vi "Getting Started - External Memory (FPGA).vi"() -> ()   [LabVIEW 2023]
doc: "This VI demonstrates the different methods of accessing DRAM on a FLexRIO FPGA Module."
uses:
  <vilib>/Platform/TimedLoop/XDataNode/wakeup.ctl
  <vilib>/Platform/TimedLoop/XDataNode/XDNodeRunTimeDep.lvlib
  <vilib>/Platform/TimedLoop/XDataNode/nitl_modes.ctl
  <vilib>/Platform/TimedLoop/XDataNode/timing_clust.ctl
  <vilib>/Platform/TimedLoop/XDataNode/XDataNode.xnode
  <instrlib>/_niInstr/Basic Elements/v1/FPGA/niInstr Basic Elements v1 FPGA.lvlib
  <instrlib>/_niInstr/Memory/v1/FPGA/DRAM/niInstr Memory DRAM v1 FPGA.lvclass
  <vilib>/rvi/DataTransferAndStorage/Container/XNode/niFpgaContainer.xnode
  <vilib>/rvi/Memory/Memory_Emulation/niFpgaMemoryFastEmulationDramWriteAndRequestData.vi
  <vilib>/rvi/Memory/Memory_Emulation/niFpgaMemoryEmulationDramWriteAndRequestData.vi
  <instrlib>/_niInstr/Memory/v1/FPGA/Memory/Public/Write Data (With Byte Enables).ctl
  <instrlib>/_niInstr/Memory/v1/FPGA/Memory/niInstr Memory v1 FPGA.lvclass
  <instrlib>/_niInstr/Memory/v1/FPGA/Memory/Public/Read Request.ctl
  <instrlib>/_niInstr/Memory/v1/FPGA/DRAM/Public/Timeslot Arbiter Configuration.ctl
  <instrlib>/_niInstr/Data Formatting/v1/FPGA/niInstr Data Formatting v1 FPGA.lvlib
  <instrlib>/_niInstr/Data Formatting/v1/FPGA/Private/Convert/U64 array to Boolean Array.vi
  <instrlib>/_niInstr/Data Formatting/v1/FPGA/Private/Convert/Boolean Array to U64 Array.vi
  <instrlib>/_niInstr/Memory/v1/FPGA/DRAM U64/Public/Create.vi
  <instrlib>/_niInstr/Memory/v1/FPGA/DRAM U64/niInstr Memory DRAM U64 v1 FPGA.lvclass
  <instrlib>/_niInstr/Memory/v1/FPGA/DRAM U128/Public/Create.vi
  <instrlib>/_niInstr/Memory/v1/FPGA/DRAM U128/niInstr Memory DRAM U128 v1 FPGA.lvclass
  <instrlib>/_niInstr/Memory/v1/FPGA/DRAM U512/Public/Create.vi
  <instrlib>/_niInstr/Memory/v1/FPGA/DRAM U512/niInstr Memory DRAM U512 v1 FPGA.lvclass
  <instrlib>/_niInstr/Basic Elements/v1/FPGA/Private/Write U32 FIFO.vi
  <instrlib>/_niInstr/Basic Elements/v1/FPGA/Private/Read U32 FIFO.vi
  <instrlib>/FlexRIO/DRAM FIFO/v2/FPGA/DRAM FIFO/DRAM FIFO v2 FPGA.lvclass
  <instrlib>/FlexRIO/DRAM FIFO/v2/FPGA/DRAM FIFO/Private/DRAM FIFO U512/Create 512x1 DRAM FIFO.vi
  <instrlib>/FlexRIO/DRAM FIFO/v2/FPGA/DRAM FIFO/Private/DRAM FIFO U512/DRAM FIFO U512 v2 FPGA.lvclass
  <instrlib>/FlexRIO/DRAM FIFO/v2/FPGA/DRAM FIFO/FIFO Depth.ctl
  <instrlib>/FlexRIO/DRAM FIFO/v2/FPGA/DRAM FIFO/Private/DRAM FIFO U64/Create 64x1 DRAM FIFO.vi
  <instrlib>/FlexRIO/DRAM FIFO/v2/FPGA/DRAM FIFO/Private/DRAM FIFO U64/DRAM FIFO U64 v2 FPGA.lvclass
  <instrlib>/FlexRIO/DRAM FIFO/v2/FPGA/DRAM FIFO/Private/DRAM FIFO U128/Create 128x1 DRAM FIFO.vi
  <instrlib>/FlexRIO/DRAM FIFO/v2/FPGA/DRAM FIFO/Private/DRAM FIFO U128/DRAM FIFO U128 v2 FPGA.lvclass
  <instrlib>/FlexRIO/DRAM FIFO/v2/FPGA/DRAM FIFO/Pack U32.vi
  <instrlib>/FlexRIO/DRAM FIFO/v2/FPGA/DRAM FIFO/Unpack U8.vi
  <vilib>/rvi/Memory/Memory_Emulation/niFpgaMemoryEmulationDramRetrieveData.vi
  <instrlib>/_niInstr/Memory/v1/FPGA/DRAM U256/Public/Create.vi
  <instrlib>/_niInstr/Memory/v1/FPGA/DRAM U256/niInstr Memory DRAM U256 v1 FPGA.lvclass
  <instrlib>/FlexRIO/DRAM FIFO/v2/FPGA/DRAM FIFO/Private/DRAM FIFO U256/Create 256x1 DRAM FIFO.vi
  <instrlib>/FlexRIO/DRAM FIFO/v2/FPGA/DRAM FIFO/Private/DRAM FIFO U256/DRAM FIFO U256 v2 FPGA.lvclass
  <instrlib>/FlexRIO/DRAM FIFO/v2/FPGA/DRAM FIFO/DRAM FIFO Status.ctl
panel:
  out "DRAM FIFO Status":T1
  out "elements per valid output":i32
  in  "DRAM FIFO - read grant time":u16=100
  in  "DRAM FIFO - write grant time":u16=100
  in  "Memory IDL - Write Data":u64[](array[numeric])=[0, 0, 0, 0, 0, 0, 0, 0]
  out "Memory Primitive - Retrieved Data":u64
  in  "Memory Primitive - Request Valid":bool
  in  "Memory Primitive - Request Address":u32
  out "Memory IDL - Retrieved Data":u64[](array[numeric])
  in  "Memory IDL - read grant time":u16
  in  "Memory IDL - write grant time":u16
  in  "Memory IDL - Request Valid":bool
  in  "Memory IDL - Request Address":u32
  in  "Memory IDL - Write Valid":bool
  in  "Memory IDL - Write Address":u32
  in  "Memory Primitive - Write Valid":bool=TRUE
  in  "Memory Primitive - Write Data":u64
  in  "Memory Primitive - Write Address":u32
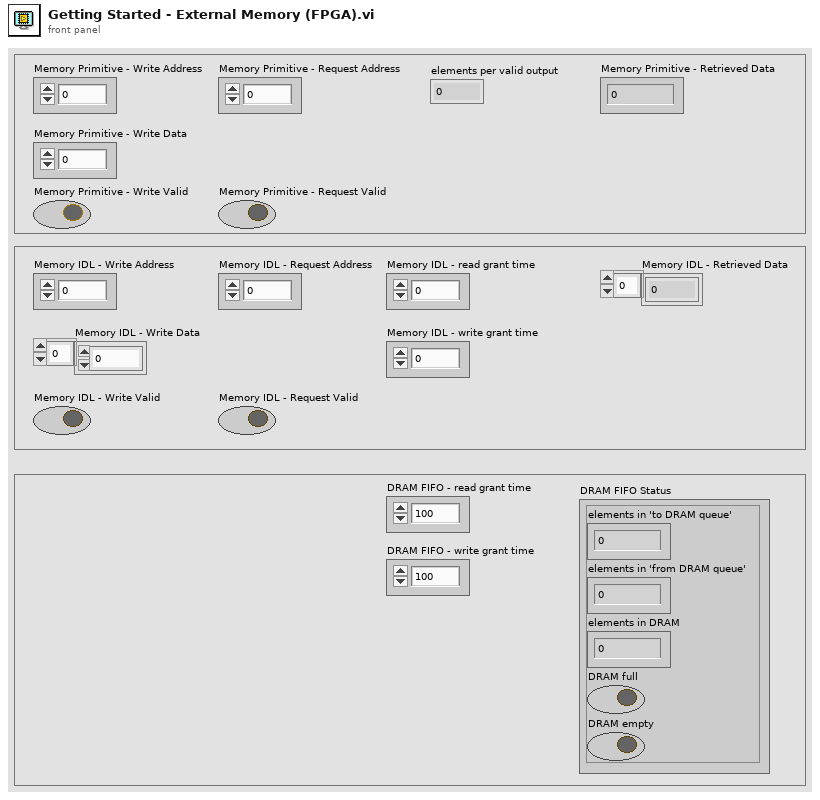
[diagram p1: front panel]
types:
  T1 = typedef "DRAM FIFO v2 FPGA.lvclass/DRAM FIFO Status.ctl" = cluster{"elements in 'to DRAM queue'":u32, "elements in 'from DRAM queue'":u32, "elements in DRAM":u32, "DRAM full":bool, "DRAM empty":bool}
  T2 = typedef "DRAM FIFO v2 FPGA.lvclass/FIFO Depth.ctl" = u8
  T3 = typedef "XDNodeRunTimeDep.lvlib/timing_clust.ctl" = cluster{"Expected End [f-1]":u64, "Actual End [f-1]":u64, "Finished Late? [f-1]":bool, "Expected End [i-1]":u64, "Actual End [i-1]":u64, "Finished Late? [i-1]":bool, "Expected Start [i]":u64, "Actual Start [i]":u64, "Expected Start [f]":u64, "Actual Start [f]":u64, "Source Name":string, "Structure Name":string, "Period":i64, "Deadline":i64, "Offset":i64, "Start":i64, "Priority":i32, "Timeout":i32, "Mode":T4, "Wakeup Reason":T5, "Error":errorcluster, "Source Type":string, "Secondary Source Type":string, "Global End Time":u64, "Global Start Time":u64, "Frame Duration":u64, "Iteration Duration":u64, "Assigned CPU":i32, "I/O Scan Engine Mode":u32}
  T4 = typedef "XDNodeRunTimeDep.lvlib/nitl_modes.ctl" = enum32{"No Change", "Process missed periods, maintain original phase", "Discard missed periods, maintain original phase", "Process missed periods, ignore original phase", "Discard missed periods, ignore original phase"}
  T5 = typedef "XDNodeRunTimeDep.lvlib/wakeup.ctl" = enum32{"Normal", "Aborted", "Asynchronous wakeup", "Timing source error", "Timed loop error", "Timeout"}
  T6 = typedef "niInstr Memory DRAM v1 FPGA.lvclass/Timeslot Arbiter Configuration.ctl" = cluster{"write grant time (clocks)":u16, "read grant time (clocks)":u16}
  T7 = typedef "niInstr Memory v1 FPGA.lvclass/Read Request.ctl" = cluster{"address":u32, "valid":bool}
  T8 = typedef "niInstr Memory v1 FPGA.lvclass/Write Data (With Byte Enables).ctl" = cluster{"address":u32, "data":bool[], "byte enables":bool[], "valid":bool}
  T9 = typedef "niInstr Memory v1 FPGA.lvclass/Retrieve Data.ctl" = cluster{"data":bool[], "valid":bool}
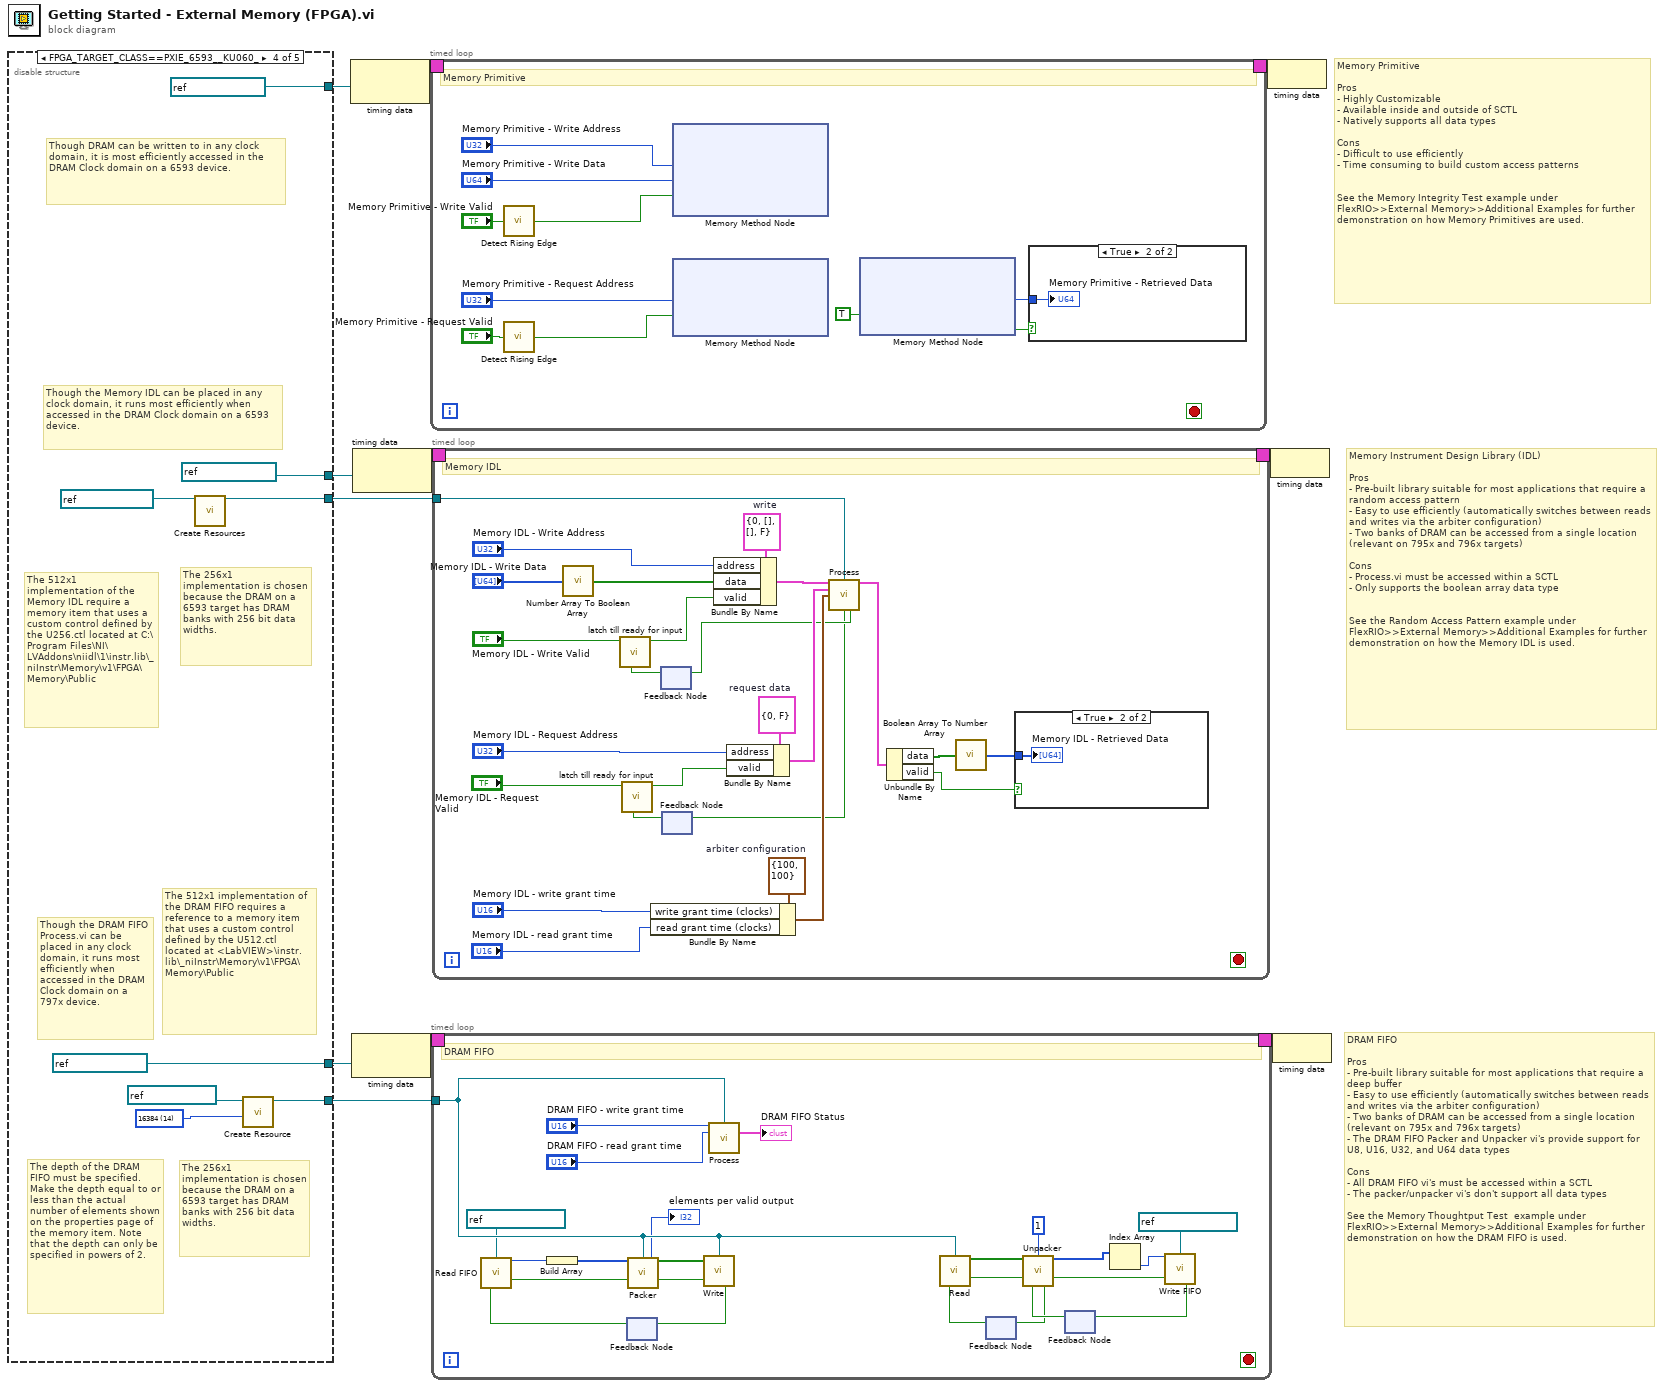
[diagram p0: block diagram]
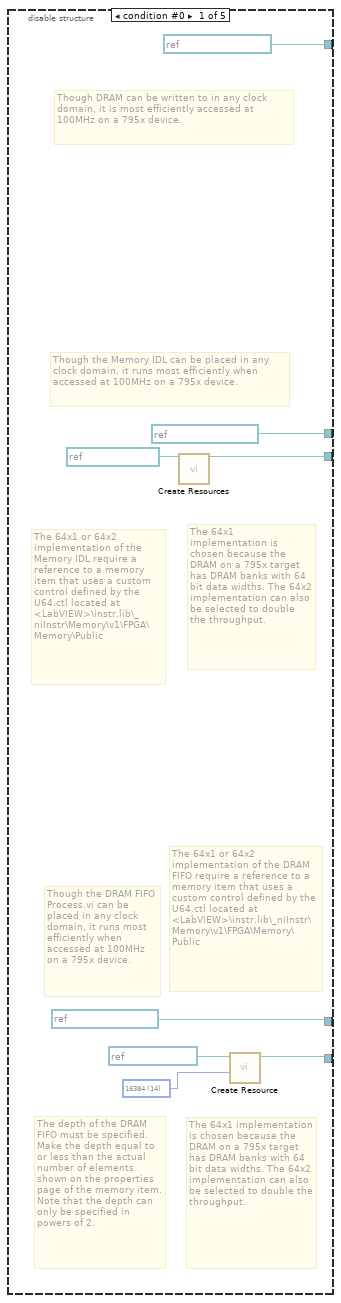
[diagram p4: hidden frame]
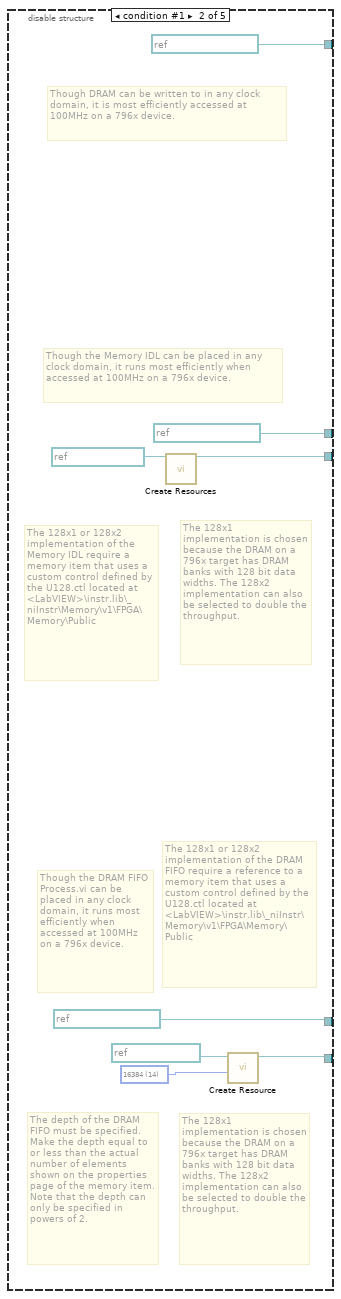
[diagram p5: hidden frame]
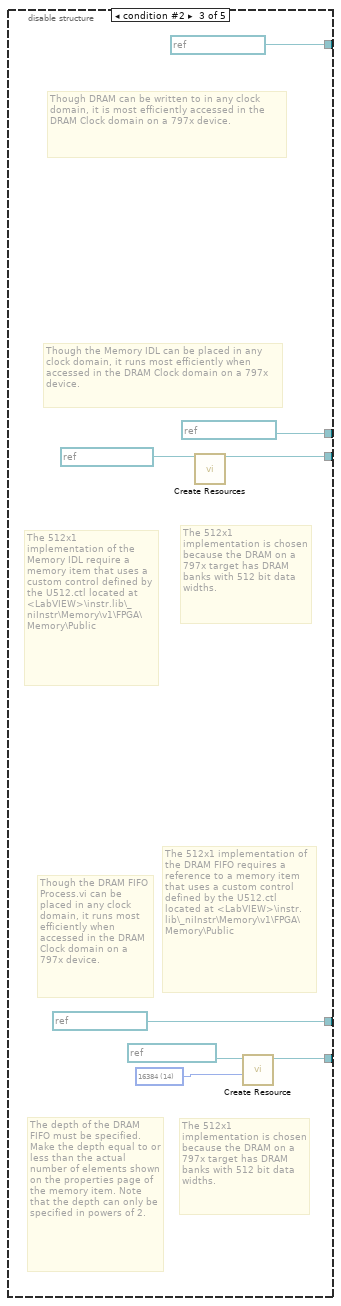
[diagram p6: hidden frame]
diagram:
  # "DRAM FIFO\n\nPros\n- Pre-built library suitable for most applications that require a deep buffer\n- Easy to use efficiently (automatically switches between reads and writes via the arbiter configuration)\n- Two banks of DRAM can be accessed from a single location (relevant on 795x and 796x targets)\n- The DRAM FIFO Packer and Unpacker vi's provide support for U8, U16, U32, and U64 data types\n\nCons\n- All DRAM FIFO vi's must be accessed within a SCTL\n- The packer/unpacker vi's don't support all data types\n\nSee the Memory Thoughtput Test  example under FlexRIO>>External Memory>>Additional Examples for further demonstration on how the DRAM FIFO is used."
  # "Memory Instrument Design Library (IDL)\n\nPros\n- Pre-built library suitable for most applications that require a random access pattern \n- Easy to use efficiently (automatically switches between reads and writes via the arbiter configuration)\n- Two banks of DRAM can be accessed from a single location (relevant on 795x and 796x targets)\n\nCons\n- Process.vi must be accessed within a SCTL\n- Only supports the boolean array data type\n\n\nSee the Random Access Pattern example under FlexRIO>>External Memory>>Additional Examples for further demonstration on how the Memory IDL is used."
  # "Memory Primitive \n\nPros\n- Highly Customizable\n- Available inside and outside of SCTL\n- Natively supports all data types\n\nCons\n- Difficult to use efficiently\n- Time consuming to build custom access patterns\n\n\nSee the Memory Integrity Test example under FlexRIO>>External Memory>>Additional Examples for further demonstration on how Memory Primitives are used."
  n1 = disable-structure shown="FPGA_TARGET_CLASS==PXIE_6593__KU060_" {
    disable-tunnel: [w16 w27 w34 w43 _] -> w7
    disable-tunnel: [refnum<k21> "100 MHz Clock" ("Source Name") refnum<k21> "100 MHz Clock" ("Source Name") refnum<k21> "DRAM Clock" ("Source Name") refnum<k21> "DRAM Clock" ("Source Name") _] -> w4
    disable-tunnel: [refnum<k21> "100 MHz Clock" ("Source Name") refnum<k21> "100 MHz Clock" ("Source Name") refnum<k21> "DRAM Clock" ("Source Name") refnum<k21> "DRAM Clock" ("Source Name") _] -> w3
    disable-tunnel: [refnum<k21> "100 MHz Clock" ("Source Name") refnum<k21> "100 MHz Clock" ("Source Name") refnum<k21> "DRAM Clock" ("Source Name") refnum<k21> "DRAM Clock" ("Source Name") _] -> w2
    disable-tunnel: [w12 w20 w28 w37 _] -> w1
    frame condition #0 {
      w15 = T2 14 items=["4"=2, "8"=3, "16"=4, "32"=5, "64"=6, "128"=7, "256"=8, "512"=9, "1024"=10, "2048"=11, "4096"=12, "8192"=13, "16384"=14, "32768"=15, "65536"=16, "131072"=17, "262144"=18, "524288"=19, "1048576"=20, "2097152"=21, "4194304"=22, "8388608"=23, "16777216"=24, "33554432"=25, "67108864"=26, "134217728"=27, "268435456"=28, "536870912"=29, "1073741824"=30, "2147483648"=31, "4294967296"=32] ("Actual # of DRAM Elements")
      # "The depth of the DRAM FIFO must be specified. Make the depth equal to or less than the actual number of elements shown on the properties page of the memory item. Note that the depth can only be specified in powers of 2."
      # "The 64x1 implementation is chosen because the DRAM on a 795x target has DRAM banks with 64 bit data widths. The 64x2 implementation can also be selected to double the throughput."
      # "The 64x1 or 64x2 implementation of the DRAM FIFO require a reference to a memory item that uses a custom control defined by the U64.ctl located at <LabVIEW>\\instr.lib\\_niInstr\\Memory\\v1\\FPGA\\Memory\\Public"
      # "Though the DRAM FIFO Process.vi can be placed in any clock domain, it runs most efficiently when  accessed at 100MHz on a 795x device."
      # "The 64x1 implementation is chosen because the DRAM on a 795x target has DRAM banks with 64 bit data widths. The 64x2 implementation can also be selected to double the throughput."
      # "The 64x1 or 64x2  implementation of the Memory IDL require a reference to a memory item that uses a custom control defined by the U64.ctl located at <LabVIEW>\\instr.lib\\_niInstr\\Memory\\v1\\FPGA\\Memory\\Public"
      # "Though the Memory IDL can be placed in any clock domain, it runs most efficiently when  accessed at 100MHz on a 795x device."
      # "Though DRAM can be written to in any clock domain, it is most efficiently accessed at 100MHz on a 795x device."
      n2 = call-poly <instrlib>:"Create Resources.vi"("memory in"=refnum<k21> "Memory IDL") -> ("memory out"=w16:refnum<class "niInstr Memory DRAM U64 v1 FPGA.lvclass">)  [unwired: 14 in]
      n3 = call-poly <instrlib>:"Create Resource.vi"("actual # of DRAM elements"=w15, "memory refnum"=refnum<k21> "DRAM FIFO" ("Memory Refnum")) -> ("DRAM FIFO ref out"=w12:refnum<class "DRAM FIFO v2 FPGA.lvclass">)  [unwired: 9 in]
    }
    frame condition #1 {
      w23 = T2 14 items=["4"=2, "8"=3, "16"=4, "32"=5, "64"=6, "128"=7, "256"=8, "512"=9, "1024"=10, "2048"=11, "4096"=12, "8192"=13, "16384"=14, "32768"=15, "65536"=16, "131072"=17, "262144"=18, "524288"=19, "1048576"=20, "2097152"=21, "4194304"=22, "8388608"=23, "16777216"=24, "33554432"=25, "67108864"=26, "134217728"=27, "268435456"=28, "536870912"=29, "1073741824"=30, "2147483648"=31, "4294967296"=32] ("Actual # of DRAM Elements")
      # "The depth of the DRAM FIFO must be specified. Make the depth equal to or less than the actual number of elements shown on the properties page of the memory item. Note that the depth can only be specified in powers of 2."
      # "The 128x1 implementation is chosen because the DRAM on a 796x target has DRAM banks with 128 bit data widths. The 128x2 implementation can also be selected to double the throughput."
      # "The 128x1 or 128x2  implementation of the DRAM FIFO require a reference to a memory item that uses a custom control defined by the U128.ctl located at <LabVIEW>\\instr.lib\\_niInstr\\Memory\\v1\\FPGA\\Memory\\Public"
      # "Though the DRAM FIFO Process.vi can be placed in any clock domain, it runs most efficiently when  accessed at 100MHz on a 796x device."
      # "The 128x1 implementation is chosen because the DRAM on a 796x target has DRAM banks with 128 bit data widths. The 128x2 implementation can also be selected to double the throughput."
      # "The 128x1 or 128x2 implementation of the Memory IDL require a memory item that uses a custom control defined by the U128.ctl located at <LabVIEW>\\instr.lib\\_niInstr\\Memory\\v1\\FPGA\\Memory\\Public"
      # "Though the Memory IDL can be placed in any clock domain, it runs most efficiently when  accessed at 100MHz on a 796x device."
      # "Though DRAM can be written to in any clock domain, it is most efficiently accessed at 100MHz on a 796x device."
      n4 = call-poly <instrlib>:"Create Resources.vi"("memory in"=refnum<k21> "Memory IDL") -> ("memory out"=w27:refnum<class "niInstr Memory DRAM U128 v1 FPGA.lvclass">)  [unwired: 14 in]
      n5 = call-poly <instrlib>:"Create Resource.vi"("actual # of DRAM elements"=w23, "memory refnum"=refnum<k21> "DRAM FIFO" ("Memory Refnum")) -> ("DRAM FIFO ref out"=w20:refnum<class "DRAM FIFO v2 FPGA.lvclass">)  [unwired: 9 in]
    }
    frame condition #2 {
      w31 = T2 14 items=["4"=2, "8"=3, "16"=4, "32"=5, "64"=6, "128"=7, "256"=8, "512"=9, "1024"=10, "2048"=11, "4096"=12, "8192"=13, "16384"=14, "32768"=15, "65536"=16, "131072"=17, "262144"=18, "524288"=19, "1048576"=20, "2097152"=21, "4194304"=22, "8388608"=23, "16777216"=24, "33554432"=25, "67108864"=26, "134217728"=27, "268435456"=28, "536870912"=29, "1073741824"=30, "2147483648"=31, "4294967296"=32] ("Actual # of DRAM Elements")
      # "The depth of the DRAM FIFO must be specified. Make the depth equal to or less than the actual number of elements shown on the properties page of the memory item. Note that the depth can only be specified in powers of 2."
      # "The 512x1 implementation is chosen because the DRAM on a 797x target has DRAM banks with 512 bit data widths."
      # "The 512x1 implementation of the DRAM FIFO requires a reference to a memory item that uses a custom control defined by the U512.ctl located at <LabVIEW>\\instr.lib\\_niInstr\\Memory\\v1\\FPGA\\Memory\\Public"
      # "Though the DRAM FIFO Process.vi can be placed in any clock domain, it runs most efficiently when accessed in the DRAM Clock domain on a 797x device."
      # "The 512x1 implementation is chosen because the DRAM on a 797x target has DRAM banks with 512 bit data widths."
      # "The 512x1 implementation of the Memory IDL require a memory item that uses a custom control defined by the U512.ctl located at <LabVIEW>\\instr.lib\\_niInstr\\Memory\\v1\\FPGA\\Memory\\Public"
      # "Though the Memory IDL can be placed in any clock domain, it runs most efficiently when  accessed in the DRAM Clock domain on a 797x device."
      # "Though DRAM can be written to in any clock domain, it is most efficiently accessed in the DRAM Clock domain on a 797x device."
      n6 = call-poly <instrlib>:"Create Resources.vi"("memory in"=refnum<k21> "Memory IDL") -> ("memory out"=w34:refnum<class "niInstr Memory DRAM U512 v1 FPGA.lvclass">)  [unwired: 14 in]
      n7 = call-poly <instrlib>:"Create Resource.vi"("actual # of DRAM elements"=w31, "memory refnum"=refnum<k21> "DRAM FIFO" ("Memory In")) -> ("DRAM FIFO ref out"=w28:refnum<class "DRAM FIFO v2 FPGA.lvclass">)  [unwired: 9 in]
    }
    frame condition #3 (active) {
      w40 = T2 14 items=["4"=2, "8"=3, "16"=4, "32"=5, "64"=6, "128"=7, "256"=8, "512"=9, "1024"=10, "2048"=11, "4096"=12, "8192"=13, "16384"=14, "32768"=15, "65536"=16, "131072"=17, "262144"=18, "524288"=19, "1048576"=20, "2097152"=21, "4194304"=22, "8388608"=23, "16777216"=24, "33554432"=25, "67108864"=26, "134217728"=27, "268435456"=28, "536870912"=29, "1073741824"=30, "2147483648"=31, "4294967296"=32] ("Actual # of DRAM Elements")
      # "The depth of the DRAM FIFO must be specified. Make the depth equal to or less than the actual number of elements shown on the properties page of the memory item. Note that the depth can only be specified in powers of 2."
      # "The 256x1 implementation is chosen because the DRAM on a 6593 target has DRAM banks with 256 bit data widths."
      # "The 512x1 implementation of the DRAM FIFO requires a reference to a memory item that uses a custom control defined by the U512.ctl located at <LabVIEW>\\instr.lib\\_niInstr\\Memory\\v1\\FPGA\\Memory\\Public"
      # "Though the DRAM FIFO Process.vi can be placed in any clock domain, it runs most efficiently when accessed in the DRAM Clock domain on a 797x device."
      # "The 256x1 implementation is chosen because the DRAM on a 6593 target has DRAM banks with 256 bit data widths."
      # "The 512x1 implementation of the Memory IDL require a memory item that uses a custom control defined by the U256.ctl located at C:\\Program Files\\NI\\LVAddons\\niidl\\1\\instr.lib\\_niInstr\\Memory\\v1\\FPGA\\Memory\\Public"
      # "Though the Memory IDL can be placed in any clock domain, it runs most efficiently when  accessed in the DRAM Clock domain on a 6593 device."
      # "Though DRAM can be written to in any clock domain, it is most efficiently accessed in the DRAM Clock domain on a 6593 device."
      n8 = call-poly <instrlib>:"Create Resources.vi"("memory in"=refnum<k21> "Memory IDL") -> ("memory out"=w43:refnum<class "niInstr Memory DRAM U256 v1 FPGA.lvclass">)  [unwired: 14 in]
      n9 = call-poly <instrlib>:"Create Resource.vi"("actual # of DRAM elements"=w40, "memory refnum"=refnum<k21> "DRAM FIFO" ("Memory In")) -> ("DRAM FIFO ref out"=w37:refnum<class "DRAM FIFO v2 FPGA.lvclass">)  [unwired: 9 in]
    }
    frame condition #4 {
      # "#todo add fail compile VI (where is it?)"
    }
  }
  n10 = node-c288(w4) -> (w6:T3)
  n11 = node-c288(w2) -> (w11:T3)
  n12 = node-c288(w3) -> (w9:T3)
  n13 = timed-loop {
    timing: w6 -> [_]
    timing-out: [_] -> w5
    stop <- _ stop-if-true
    # "Memory Primitive"
    n14 = call <instrlib>:"Detect Rising Edge.vi"("signal"="Memory Primitive - Write Valid") -> ("edge detected"=w50:bool)  [unwired: 14 in]
    n15 = call <instrlib>:"Detect Rising Edge.vi"("signal"="Memory Primitive - Request Valid") -> ("edge detected"=w44:bool)  [unwired: 14 in]
    n16 = xnode ("Memory Method Node")("Address"="Memory Primitive - Write Address", "Data"="Memory Primitive - Write Data", "Input Valid"=w50) -> ()  [unwired: 2 in, 3 out]
    n17 = xnode ("Memory Method Node")("Address"="Memory Primitive - Request Address", "Input Valid"=w44) -> ()  [unwired: 1 in, 2 out]
    n18 = xnode ("Memory Method Node")("Ready for Output"=TRUE) -> ("Data"=w48:u64, "Output Valid"=w47:bool)  [unwired: 1 in, 1 out]
    n19 = case shown="True" w47 {
      tunnel: w48 -> [_ w54]
      frame False {
      }
      frame True {
        "Memory Primitive - Retrieved Data" <- w54
      }
    }
  }
  n20 = timed-loop {
    timing: w11 -> [_]
    timing-out: [_] -> w10
    tunnel: w1 -> [w69]
    stop <- _ stop-if-true
    # "DRAM FIFO"
    n21 = feedback #1() -> (w65:bool)  [unwired: 1 in]
    n22 = call-poly <instrlib>:"Read FIFO.vi"("fifo"=refnum<k21> "HostToTarget", "ready for output"=w65) -> ("output data"=w73:u32, "output valid"=w68:bool)  [unwired: 12 in]
    n23 = Build Array(w73) -> (w72:u32[])
    n24 = call-poly <instrlib>:"Packer.vi"("data in"=w72, "DRAM FIFO in"=w69, "input valid"=w68) -> ("elements per valid output"=→"elements per valid output":i32, "data out"=w70:bool[], "output valid"=w71:bool)  [unwired: 10 in]
    n25 = call <instrlib>:"Write.vi"("element"=w70, "DRAM FIFO ref in"=w69, "input valid"=w71) -> ("ready for input"=w66:bool)  [unwired: 12 in]
    n26 = feedback-in #1(w66) -> ()
    n27 = call <instrlib>:"Process.vi"("write grant time (clock ticks)"="DRAM FIFO - write grant time", "DRAM FIFO ref in"=w69, "read grant time (clock ticks)"="DRAM FIFO - read grant time") -> ("status"=→"DRAM FIFO Status":T1)  [unwired: 11 in, 1 out]
    n28 = feedback #2() -> (w61:bool)  [unwired: 1 in]
    n29 = call <instrlib>:"Read.vi"("DRAM FIFO ref in"=w69, "ready for output"=w61) -> ("element"=w78:bool[], "output valid"=w77:bool)  [unwired: 12 in]
    n30 = feedback #3() -> (w63:bool)  [unwired: 1 in]
    n31 = call-poly <instrlib>:"Unpacker.vi"("packed data in"=w78, "output data size (elements)"=u16 1, "input valid"=w77, "ready for output"=w63) -> ("unpacked data out"=w76:u8[], "output valid"=w74:bool, "ready for input"=w62:bool)  [unwired: 9 in]
    n32 = feedback-in #2(w62) -> ()
    n33 = Index Array(array=w76) -> (element=w75:u8)  [unwired: 1 in]
    n34 = call-poly <instrlib>:"Write FIFO.vi"("input data"=w75, "fifo"=refnum<k21> "TargetToHost", "input valid"=w74) -> ("ready for input"=w64:bool)  [unwired: 12 in]
    n35 = feedback-in #3(w64) -> ()
  }
  n36 = timed-loop {
    timing: w9 -> [_]
    timing-out: [_] -> w8
    tunnel: w7 -> [w107]
    stop <- _ stop-if-true
    w103 = T6 {"write grant time (clocks)"=100, "read grant time (clocks)"=100}  # arbiter configuration
    w102 = T7 {"address"=0, "valid"=FALSE}  # request data
    w105 = T8 {"address"=0, "data"=[], "byte enables"=[], "valid"=FALSE}  # write
    # "Memory IDL"
    n37 = call-poly <instrlib>:"Number Array To Boolean Array.vi"("data in"="Memory IDL - Write Data") -> ("data out"=w93:bool[])  [unwired: 14 in]
    n38 = Bundle By Name(cluster=w103, "write grant time (clocks)"="Memory IDL - write grant time", "read grant time (clocks)"="Memory IDL - read grant time") -> (w100:T6)
    n39 = feedback #4() -> (w89:bool)  [unwired: 1 in]
    n40 = call "latch till ready for input.vi"("Ready for Output"=w89, "Request Valid"="Memory IDL - Write Valid") -> ("output valid"=w84:bool)  [unwired: 9 in]
    n41 = feedback #5() -> (w87:bool)  [unwired: 1 in]
    n42 = call "latch till ready for input.vi"("Ready for Output"=w87, "Request Valid"="Memory IDL - Request Valid") -> ("output valid"=w86:bool)  [unwired: 9 in]
    n43 = Bundle By Name(cluster=w105, "address"="Memory IDL - Write Address", "data"=w93, "valid"=w84) -> (w104:T8)
    n44 = Bundle By Name(cluster=w102, "address"="Memory IDL - Request Address", "valid"=w86) -> (w101:T7)
    n45 = call-dynamic <instrlib>:"Process.vi"("write"=w104, "memory"=w107, "request data"=w101, "arbiter configuration"=w100) -> ("retrieve data"=w106:T9, "ready for request data"=w88:bool, "ready for write"=w90:bool)  [unwired: 8 in, 1 out]
    n46 = feedback-in #4(w90) -> ()
    n47 = feedback-in #5(w88) -> ()
    n48 = Unbundle By Name(w106) -> ("data"=w95:bool[], "valid"=w91:bool)
    n49 = call-poly <instrlib>:"Boolean Array To Number Array.vi"("data in"=w95) -> ("data out"=w94:u64[])  [unwired: 14 in]
    n50 = case shown="True" w91 {
      tunnel: w94 -> [_ w108]
      frame False {
      }
      frame True {
        "Memory IDL - Retrieved Data" <- w108
      }
    }
  }
  n51 = node-c288(w5) -> ()
  n52 = node-c288(w8) -> ()
  n53 = node-c288(w10) -> ()
